vi "NMEA_ChecksumOk.vi"(9 "Error In":errorcluster, 10 "Sentence":string="$GPGGA,000052.837,,,,,0,0,,,M,,M,,*43") -> (1 "Error Out":errorcluster, 2 "CheckSumOk?":bool)   [LabVIEW 2017, in "NMEA.lvlib"]
uses:
  Downloads/NMEA_v1.1.2 LV2014/NMEA_v1.1/NMEA.lvlib
panel:
  out "CheckSum":u8 format="%.0x"
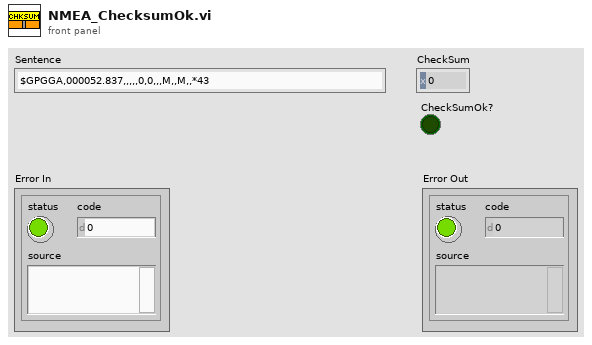
[diagram p1: front panel]
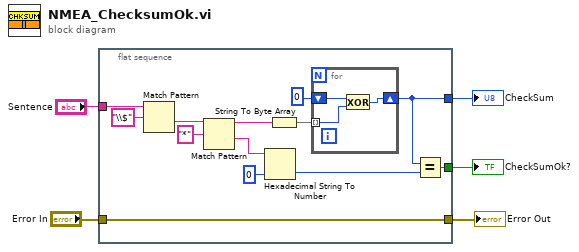
[diagram p0: block diagram]
diagram:
  n1 = flat-sequence {
    tunnel: "Sentence" -> [w16]
    tunnel: [w10] -> w4
    tunnel: [w8] -> w3
    tunnel: "Error In" -> [w6]
    tunnel: [w6] -> w1
    frame #0 {
      n2 = Match Pattern(string=w16, regular expression="\\$") -> (after substring=w13:string)  [unwired: 1 in, 3 out]
      n3 = Match Pattern(string=w13, regular expression="*") -> (before substring=w12:string, after substring=w11:string)  [unwired: 1 in, 2 out]
      n4 = Hexadecimal String To Number(string=w11, default (0uL)=u8 0 ("default (0 U32)")) -> (number=w9:u8)  [unwired: 1 in, 1 out]
      n5 = String To Byte Array(string=w12) -> (unsigned byte array=w18:u8[])
      n6 = for {
        tunnel: w18 -> [w20] mode=indexing
        shift-right: [w19] -> w10
        shift-left: u8 0 ("sum") -> [w21]
        n7 = Exclusive Or(1:w20, 2:w21) -> (0:w19:u8)
      }
      n8 = Equal?(x=w10, y=w9) -> (x = y?=w8:bool)
    }
  }
  "CheckSum" <- w4
  "CheckSumOk?" <- w3
  "Error Out" <- w1
